vi "Agileng_set.vi"(1 "VISA resource name":refnum<visa-resource-name>, 2 "Value":dbl) -> ()   [LabVIEW 2017]
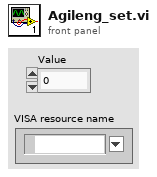
[diagram p1: front panel]
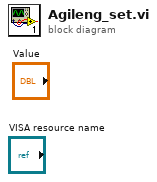
[diagram p0: block diagram]
diagram:
